vi "UIRef.vi"(8 "error in":errorcluster, 11 "Simple Sequencer TBM editor node in":refnum<class "Simple Sequencer TBM editor node.lvclass">) -> (0 "error out":errorcluster, 2 "VI refnum":refnum<vi>, 3 "Simple Sequencer TBM editor node out":refnum<class "Simple Sequencer TBM editor node.lvclass">)   [LabVIEW 2014, in "Simple Sequencer TBM editor node.lvclass"]
uses:
  Simple Sequencer TBM editor node.lvclass
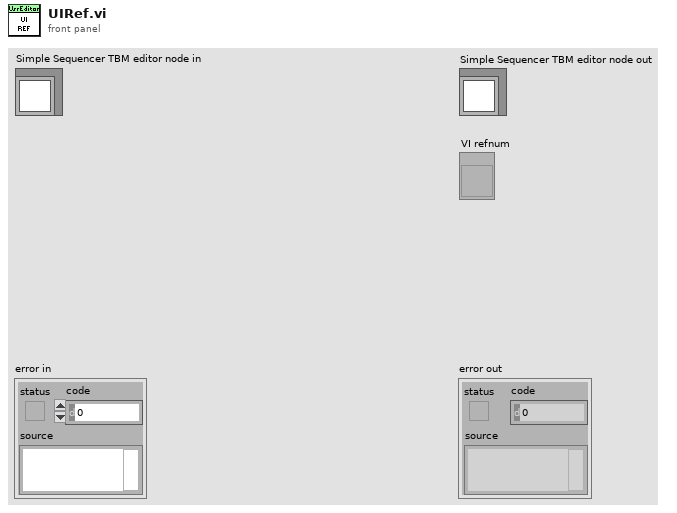
[diagram p1: front panel]
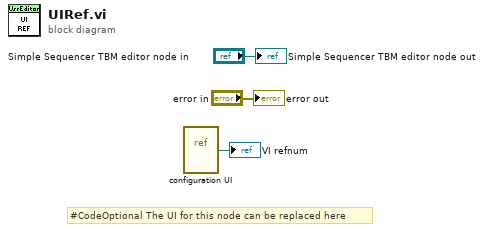
[diagram p0: block diagram]
diagram:
  # "#CodeOptional The UI for this node can be replaced here"
  n1 = vi-ref "configuration UI.vi"() -> (→"VI refnum":refnum<vi>)
  "error out" <- "error in"
  "Simple Sequencer TBM editor node out" <- "Simple Sequencer TBM editor node in"
